vi "ReadXbox.vi"(6 "Jog Speed":dbl) -> (2 "Array Jog Command":dbl[](array[numeric]))   [LabVIEW 2017]
uses:
  C:/Windows/System32/XInput9_1_0.dll
panel:
  out "Z":dbl
  out "X":dbl
  out "Y":dbl
  out "A":dbl
  out "B":dbl
  out "C":dbl
  out "RR 3":bool
  out "RR 2":bool
  out "RT":bool
  out "RL":bool
  out "RR":bool
  out "RB":bool
  out "LL":bool
  out "LR":bool
  out "LB":bool
  out "LT":bool
  out "pState 2":T1
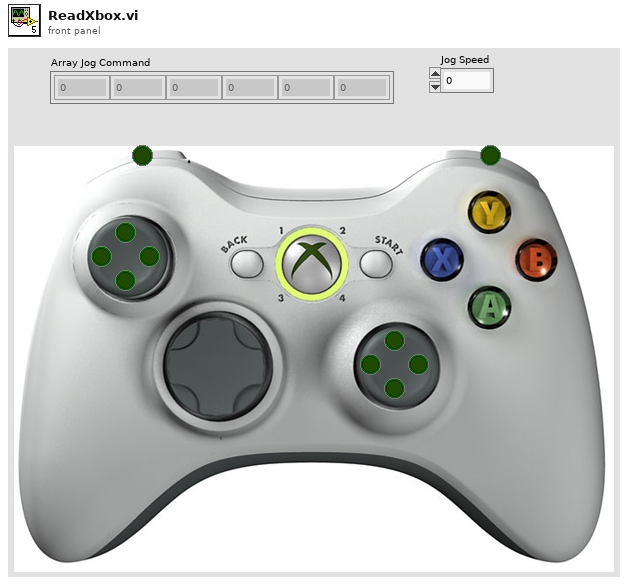
[diagram p1: front panel]
types:
  T1 = cluster{"Packet Number":u32, "Gamepad":cluster{"Buttons":u16, "Left Trigger":u8, "Right Trigger":u8, "Thumb LX":i16, "Thumb LY":i16, "Thumb RX":i16, "Thumb RY":i16}}
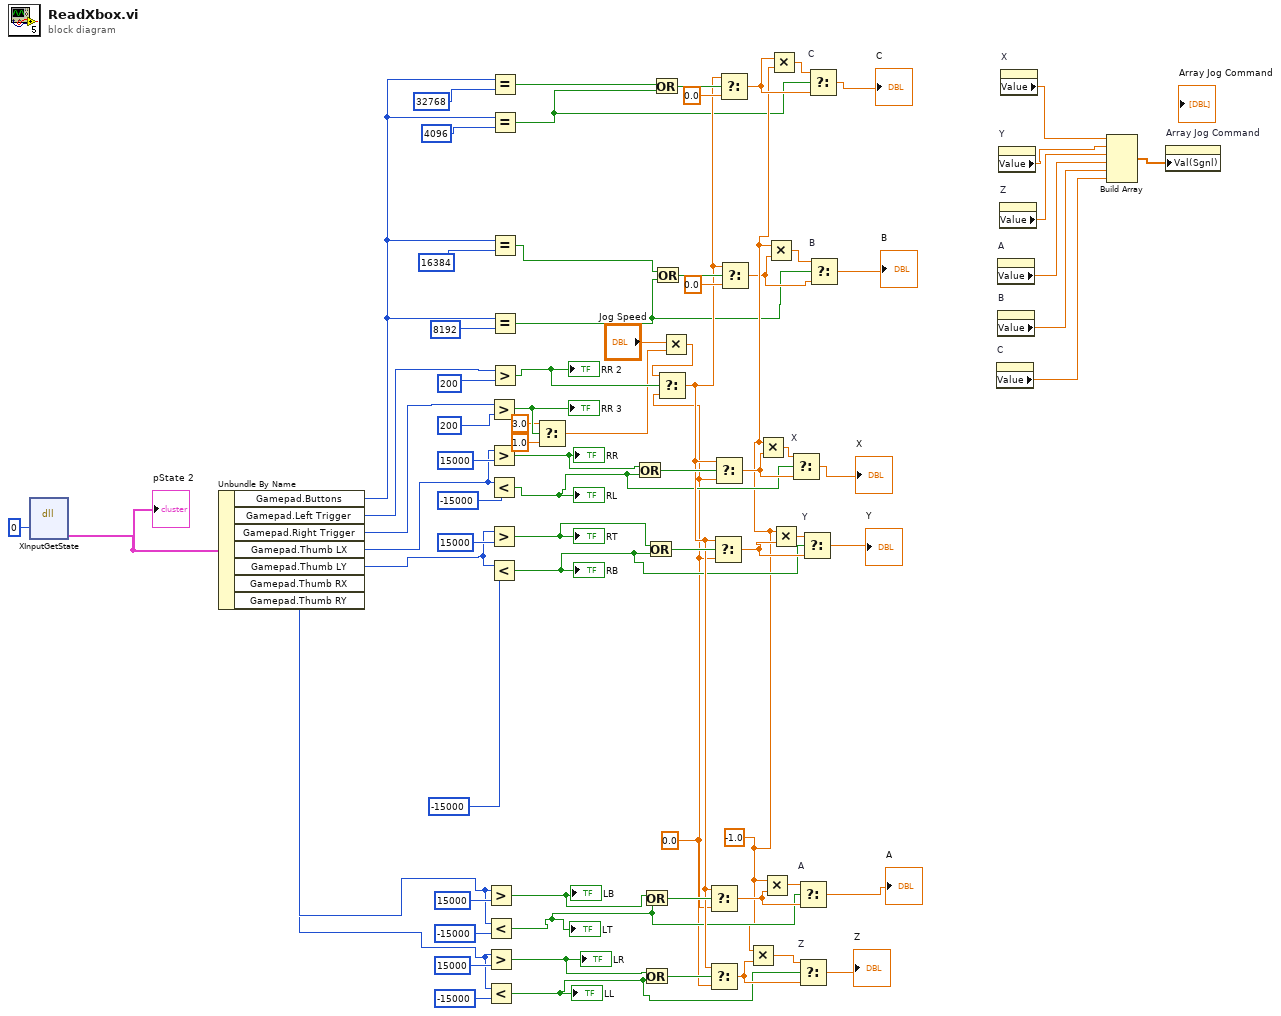
[diagram p0: block diagram]
diagram:
  w25 = -1.0 ("y")
  w28 = 0.0 ("f")
  n1 = dll-call lib="C:/Windows/System32/XInput9_1_0.dll" fn="XInputGetState"("dwUserIndex"=u32 0) -> ("pState 2"=w45:T1)  [unwired: 6 in, 2 out]
  "pState 2" <- w45
  n2 = Unbundle By Name(w45) -> ("Gamepad.Buttons"=w50:u16, "Gamepad.Left Trigger"=w67:u8, "Gamepad.Right Trigger"=w66:u8, "Gamepad.Thumb LX"=w65:i16, "Gamepad.Thumb LY"=w64:i16, "Gamepad.Thumb RX"=w63:i16, "Gamepad.Thumb RY"=w62:i16)
  n3 = Greater?(x=w63, y=15000) -> (0:w42:bool)
  "LB" <- w42
  n4 = Less?(x=w63, y=-15000) -> (x < y?=w38:bool)
  "LT" <- w38
  n5 = Greater?(x=w62, y=15000) -> (0:w41:bool)
  "LR" <- w41
  n6 = Less?(x=w62, y=-15000) -> (x < y?=w35:bool)
  "LL" <- w35
  n7 = Greater?(x=w66, y=200) -> (0:w11:bool)
  "RR 3" <- w11
  n8 = Greater?(x=w65, y=15000) -> (0:w44:bool)
  "RR" <- w44
  n9 = Less?(x=w65, y=-15000) -> (x < y?=w29:bool)
  "RL" <- w29
  n10 = Greater?(x=w64, y=15000) -> (0:w43:bool)
  "RT" <- w43
  n11 = Less?(x=w64, y=-15000) -> (x < y?=w32:bool)
  "RB" <- w32
  n12 = Equal?(x=w50, y=u16 32768) -> (x = y?=w20:bool)
  n13 = Equal?(x=w50, y=u16 4096) -> (x = y?=w22:bool)
  n14 = Equal?(x=w50, y=u16 16384) -> (x = y?=w52:bool)
  n15 = Equal?(x=w50, y=u16 8192) -> (x = y?=w21:bool)
  n16 = Greater?(x=w67, y=200) -> (0:w61:bool)
  "RR 2" <- w61
  n17 = Select(t=3.0, s=w11, f=1.0) -> (s? t:f=w8:dbl)
  n18 = Or(x=w44, y=w29) -> (x .or. y?=w60:bool)
  n19 = Or(x=w42, y=w38) -> (x .or. y?=w58:bool)
  n20 = Or(x=w41, y=w35) -> (x .or. y?=w57:bool)
  n21 = Or(x=w43, y=w32) -> (x .or. y?=w59:bool)
  n22 = Or(x=w20, y=w22) -> (x .or. y?=w54:bool)
  n23 = Or(x=w52, y=w21) -> (x .or. y?=w56:bool)
  n24 = Multiply(x="Jog Speed", y=w8) -> (x*y=w12:dbl)
  n25 = Select(t=w12, s=w61, f=w28) -> (s? t:f=w51:dbl)
  n26 = Select(t=w51, s=w58, f=w28) -> (s? t:f=w40:dbl)
  n27 = Select(t=w51, s=w57, f=w28) -> (s? t:f=w36:dbl)
  n28 = Select(t=w51, s=w59, f=w28) -> (s? t:f=w33:dbl)
  n29 = Select(t=w51, s=w60, f=w28) -> (s? t:f=w31:dbl)
  n30 = Select(t=w51, s=w54, f=0.0) -> (s? t:f=w26:dbl)
  n31 = Select(t=w51, s=w56, f=0.0) -> (s? t:f=w23:dbl)
  n32 = Multiply(x=w25, y=w36) -> (x*y=w37:dbl)
  n33 = Multiply(x=w25, y=w31) -> (x*y=w30:dbl)
  n34 = Multiply(x=w25, y=w40) -> (x*y=w39:dbl)
  n35 = Multiply(x=w25, y=w23) -> (x*y=w24:dbl)
  n36 = Multiply(x=w26, y=w25) -> (x*y=w27:dbl)
  n37 = Multiply(x=w25, y=w33) -> (x*y=w34:dbl)
  n38 = Select "X"(t=w30, s=w29, f=w31) -> (s? t:f=→"X":dbl)
  n39 = Select "A"(t=w39, s=w38, f=w40) -> (s? t:f=→"A":dbl)
  n40 = Select "Z"(t=w37, s=w35, f=w36) -> (s? t:f=→"Z":dbl)
  n41 = Select "Y"(t=w34, s=w32, f=w33) -> (s? t:f=→"Y":dbl)
  n42 = Select "C"(t=w27, s=w22, f=w26) -> (s? t:f=→"C":dbl)
  n43 = Select "B"(t=w24, s=w21, f=w23) -> (s? t:f=→"B":dbl)
  n44 = property on="C" class="DigNum (strict)"() -> ("Value"=w2:dbl)  [unwired: 2 in, 2 out]
  n45 = property on="A" class="DigNum (strict)"() -> ("Value"=w4:dbl)  [unwired: 2 in, 2 out]
  n46 = property on="B" class="DigNum (strict)"() -> ("Value"=w3:dbl)  [unwired: 2 in, 2 out]
  n47 = property on="Y" class="DigNum (strict)"() -> ("Value"=w6:dbl)  [unwired: 2 in, 2 out]
  n48 = property on="Z" class="DigNum (strict)"() -> ("Value"=w5:dbl)  [unwired: 2 in, 2 out]
  n49 = property on="X" class="DigNum (strict)"() -> ("Value"=w7:dbl)  [unwired: 2 in, 2 out]
  n50 = Build Array(w7, w6, w5, w4, w3, w2) -> (w1:dbl[])
  n51 = property on="Array Jog Command" class="Arr (strict)"("Val(Sgnl)"=w1) -> ()  [unwired: 2 in, 2 out]
